vi "Mercury iTC control RUS PGG1.vi"() -> ()   [LabVIEW 2014]
uses:
  Mercury iXX/Public/Controls/Comms Transport Layer.ctl
  itc 503 box - control.ctl
  Mercury iXX/Public/Libraries/Auxiliary/Controls/AUX Device (Read).ctl
  Mercury iXX/Public/Controls/Manufacturing Data.ctl
  Mercury iXX/Public/Libraries/Auxiliary/Controls/AUX Signals (Read).ctl
  Mercury iXX/Public/Libraries/Auxiliary/Controls/AUX Device (Set).ctl
  Mercury iXX/Public/Libraries/Auxiliary/Controls/AUX Signals (Set).ctl
  Mercury iXX/Public/Libraries/Temperature/Controls/Temperature Device (Read).ctl
  Mercury iXX/Public/Libraries/Temperature/Controls/Temperature Sensor Type.ctl
  Mercury iXX/Public/Libraries/Temperature/Controls/Excitation Cluster.ctl
  Mercury iXX/Public/Libraries/Temperature/Controls/Excitation Type.ctl
  Mercury iXX/Public/Libraries/Temperature/Controls/Calibration Cluster.ctl
  Mercury iXX/Public/Libraries/Temperature/Controls/Calibration Interpolation.ctl
  Mercury iXX/Public/Libraries/Temperature/Controls/Loop Cluster.ctl
  Mercury iXX/Public/Libraries/Temperature/Controls/Temperature Signals Cluster.ctl
  itc 503 box state.ctl
  Mercury iXX/Public/Libraries/Heater/Controls/Heater Device (Set).ctl
  Mercury iXX/Public/Libraries/Heater/Controls/Heater Signals Cluster.ctl
  Mercury iXX/Public/Libraries/Heater/Controls/Heater Device (Read).ctl
  Mercury iXX/Public/Controls/Response String.ctl
  Mercury iXX/Public/Controls/ISOBus Address.ctl
  Mercury iXX/Public/Controls/Unit String.ctl
  Mercury iXX/Public/Libraries/Auxiliary/Open/Open Auxiliary Device.vi
  Mercury iXX/Public/Libraries/Auxiliary/Configuration/Read/Aux Device (Read).vi
  Mercury iXX/Public/Libraries/Auxiliary/Configuration/Set/Aux Device (Set).vi
  Mercury iXX/Public/Libraries/Temperature/Open/Open Temperature Device.vi
  Mercury iXX/Public/Libraries/Temperature/Configuration/Read/Temperature Device (Read).vi
  Mercury iXX/Public/Libraries/Control Loop/Configuration/Set/Temperature Setpoint (Set).vi
  Mercury iXX/Public/Libraries/Control Loop/Configuration/Set/Heater Auto (Set).vi
  Mercury iXX/Public/Libraries/Heater/Open/Open Heater Device.vi
  Mercury iXX/Public/Libraries/Heater/Configuration/Read/Heater Device (Read).vi
  Mercury iXX/Public/Libraries/Heater/Configuration/Set/Heater Device (Set).vi
  Mercury iXX/Public/Libraries/Heater/Signals/Read/Voltage (Read).vi
  Mercury iXX/Public/Libraries/Control Loop/Configuration/Read/Temperature Setpoint (Read).vi
  Mercury iXX/Public/Libraries/Control Loop/Configuration/Read/PID (Read).vi
  Mercury iXX/Public/Libraries/Control Loop/Configuration/Set/P Value (Set).vi
  Mercury iXX/Public/Libraries/Control Loop/Configuration/Set/I Value (Set).vi
  Mercury iXX/Public/Libraries/Control Loop/Configuration/Set/D Value (Set).vi
  Mercury iXX/Public/Libraries/System.lvlib
  Mercury iXX/Mercury iXX.lvlib
  Mercury iXX/Public/Libraries/Temperature.lvlib
  Mercury iXX/Public/Libraries/Auxiliary.lvlib
  Mercury iXX/Public/Libraries/Control Loop.lvlib
  Mercury iXX/Public/Libraries/Heater.lvlib
panel:
  out "Response":T1
  out "itc box state OUT":T2
  out "Tab Control":T3(tab)
  out "Auxiliary Device Details":T4 {"Signals"."% Open" min=0.0 max=100.0 step=0.1 format="%.4f"; "Signals"."Position" max=20.0 step=1.0 format="%.4f"; "Speed" max=7 step=1; "Gear" max=7 step=1; "Temp V Err" min=0.0 max=20.0 step=0.1; "Temp Err" min=0.0 max=20.0 step=0.1; "Scaling Factor" min=0.0 max=99.0 step=0.1; "Min Flow" min=0.0 max=20.0 step=0.1}
  in  "Auxiliary Device":T7 {"Signals"."% Open" min=0.0 max=100.0 step=0.1 format="%#.1f"; "Speed" max=7 step=1; "Gear" max=7 step=1; "Temp V Err" min=0.0 max=20.0 step=0.1; "Temp Err" min=0.0 max=20.0 step=0.1; "Scaling Factor" min=0.0 max=99.0 step=0.1; "Min Flow" min=0.0 max=20.0 step=0.1}
  out "# of Instruments":i32
  out "Serial Number(s)":string[](array[string])
  out "T config Details":T9
  in  "T config Void":T9
  in  "Heater Device Void":T17
  out "Heater Config Details In":T19
  out "Temperature":dbl
  out "error out":errorcluster={"status"=TRUE, "code"=-1073807343, "source"="VISA Open in Mercury iXX.lvlib:System.lvlib:Open System.vi->Mercury iTC control RUS PGG1.vi"}
  in  "disable interaction with iTC":enum16{"disabled", "enabled"}(ring)
  in  "input":dbl=300.0
  in  "itc box action":T20=enum."read state"
  in  "Comms Layer":T21=enum."GPIB"
  in  "VISA resource name":refnum<visa-resource-name>="GPIB0::1::1::INSTR"
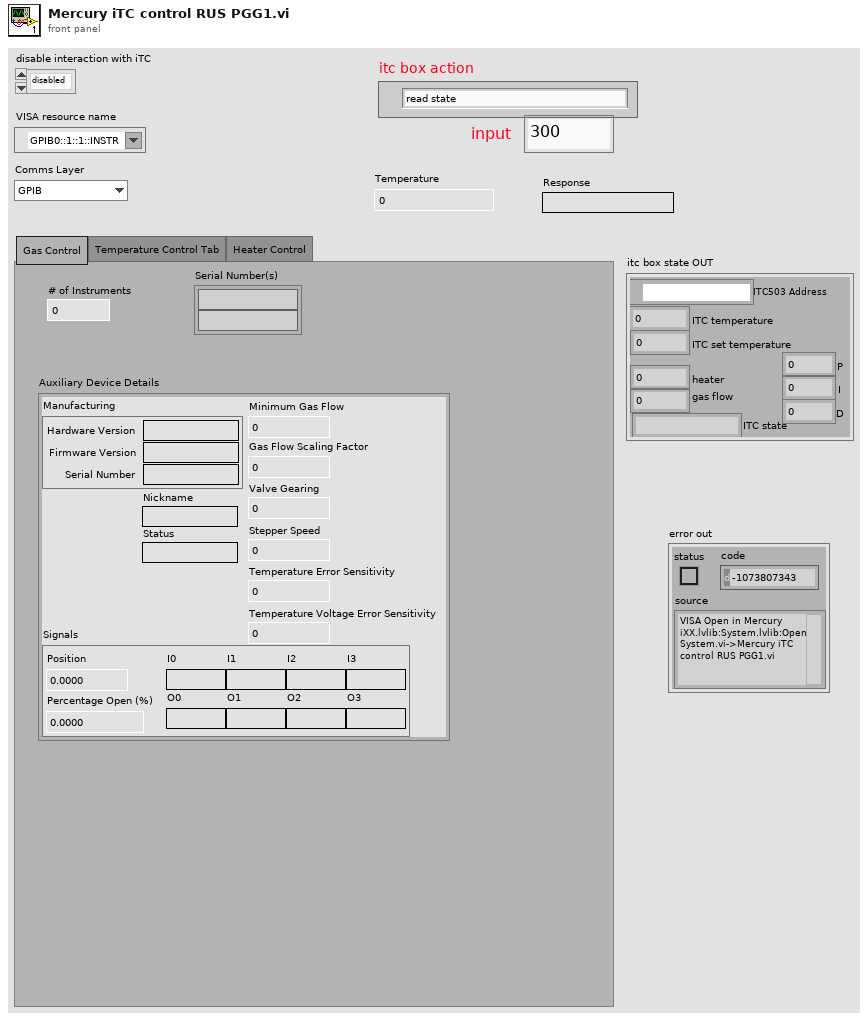
[diagram p1: front panel]
types:
  T1 = typedef "Mercury iXX.lvlib/Response String.ctl" = string
  T2 = typedef "itc 503 box state.ctl" = cluster{"ITC503 Address":refnum<visa-resource-name>, "ITC temperature":dbl, "ITC set temperature":dbl, "heater":dbl, "gas flow":dbl, "P":dbl, "D":dbl, "I":dbl, "ITC state":string, "nonzero temperature":dbl, "Magn Field (T)":dbl}
  T3 = enum32{"Gas Control", "Temperature Control Tab", "Heater Control"}
  T4 = typedef "Mercury iXX.lvlib/Auxiliary.lvlib/AUX Device (Read).ctl" = cluster{"Manufacturing":T5, "Min Flow":dbl, "Scaling Factor":dbl, "Temp Err":dbl, "Temp V Err":dbl, "Gear":u32, "Speed":u32, "Signals":T6, "Nickname":string, "Status":string}
  T5 = typedef "Mercury iXX.lvlib/Manufacturing Data.ctl" = cluster{"Hardware Version":string, "Firmware Version":string, "Serial Number":string}
  T6 = typedef "Mercury iXX.lvlib/Auxiliary.lvlib/AUX Signals (Read).ctl" = cluster{"Position":dbl, "% Open":dbl, "I0":string, "I1":string, "I2":string, "I3":string, "O0":string, "O1":string, "O2":string, "O3":string}
  T7 = typedef "Mercury iXX.lvlib/Auxiliary.lvlib/AUX Device (Set).ctl" = cluster{"Min Flow":dbl, "Scaling Factor":dbl, "Temp Err":dbl, "Temp V Err":dbl, "Gear":u32, "Speed":u32, "Signals":T8}
  T8 = typedef "Mercury iXX.lvlib/Auxiliary.lvlib/AUX Signals (Set).ctl" = cluster{"% Open":dbl}
  T9 = typedef "Mercury iXX.lvlib/Temperature.lvlib/Temperature Device (Read).ctl" = cluster{"Manufacturing":T5, "Temperature Sensor Type":T10, "Excitation":T11, "Calibration":T13, "Control Loop":T15, "Temperature Signals":T16, "Nickname":string, "Status":string}
  T10 = typedef "Mercury iXX.lvlib/Temperature.lvlib/Temperature Sensor Type.ctl" = string
  T11 = typedef "Mercury iXX.lvlib/Temperature.lvlib/Excitation Cluster.ctl" = cluster{"Excitation Type":T12, "Magnitude":string}
  T12 = typedef "Mercury iXX.lvlib/Temperature.lvlib/Excitation Type.ctl" = string
  T13 = typedef "Mercury iXX.lvlib/Temperature.lvlib/Calibration Cluster.ctl" = cluster{"Filename":string, "Interpolation":T14, "Scaling Factor":string, "Offset Factor":string, "Hot Limit":string, "Cold Limit":string, "Last Calibration":string, "Reference":string}
  T14 = typedef "Mercury iXX.lvlib/Temperature.lvlib/Calibration Interpolation.ctl" = string
  T15 = typedef "Mercury iXX.lvlib/Temperature.lvlib/Loop Cluster.ctl" = cluster{"Heater":string, "Auxiliary":string, "Heater Auto":string, "Percentage Heat":string, "Temperature Set Point":string, "PID Auto (from file)":string, "P Value":string, "I Value":string, "D Value":string, "Auto PID Table Filename":string, "Flow Auto":string, "Target Heater Table":string, "Sweep mode":string, "Sweep Table Filename":string, "Percentage Flow":string}
  T16 = typedef "Mercury iXX.lvlib/Temperature.lvlib/Temperature Signals Cluster.ctl" = cluster{"Voltage":string, "Current":string, "Power":string, "Resistance":string, "Temperature":string, "Sensitivity":string, "Reference":string}
  T17 = typedef "Mercury iXX.lvlib/Heater.lvlib/Heater Device (Set).ctl" = cluster{"Nickname":string, "Voltage Limit":string, "Nominal Resistance":string, "Maximum Power":string, "Heater Signals":T18}
  T18 = typedef "Mercury iXX.lvlib/Heater.lvlib/Heater Signals Cluster.ctl" = cluster{"Voltage":string, "Current":string, "Power":string}
  T19 = typedef "Mercury iXX.lvlib/Heater.lvlib/Heater Device (Read).ctl" = cluster{"Manufacturing":T5, "Nickname":string, "Voltage Limit":string, "Nominal Resistance":string, "Maximum Power":string, "Heater Signals":T18, "Status":string}
  T20 = typedef "itc 503 box - control.ctl" = enum16{"heater manual and zero", "heater auto", "upload D", "upload I", "upload P", "shut off", "init", "read sweep table", "disable", "enable", "read state", "set gas to", "stop sweep", "start sweep", "test", "set temperature to", "write sweep table", "-void", "set heater to"}
  T21 = typedef "Mercury iXX.lvlib/Comms Transport Layer.ctl" = enum16{"Ethernet TCP/IP", "USB", "ISOBus - RS-232", "GPIB"}
  T22 = typedef "Mercury iXX.lvlib/ISOBus Address.ctl" = i32
  T23 = typedef "Mercury iXX.lvlib/Mercury Reference.ctl" = cluster{"Comms":refnum<visa-resource-name>, "Device ID":string[], "Comms Layer":T21, "Command":string, "Query reference":T24}
  T24 = typedef "Mercury iXX.lvlib/Query Dynamic Reference.ctl" = refnum<vi>
  T25 = typedef "Mercury iXX.lvlib/Unit String.ctl" = string
  T26 = typedef "Mercury iXX.lvlib/Control Loop.lvlib/PID cluster.ctl" = cluster{"P":dbl, "I":dbl, "D":dbl}
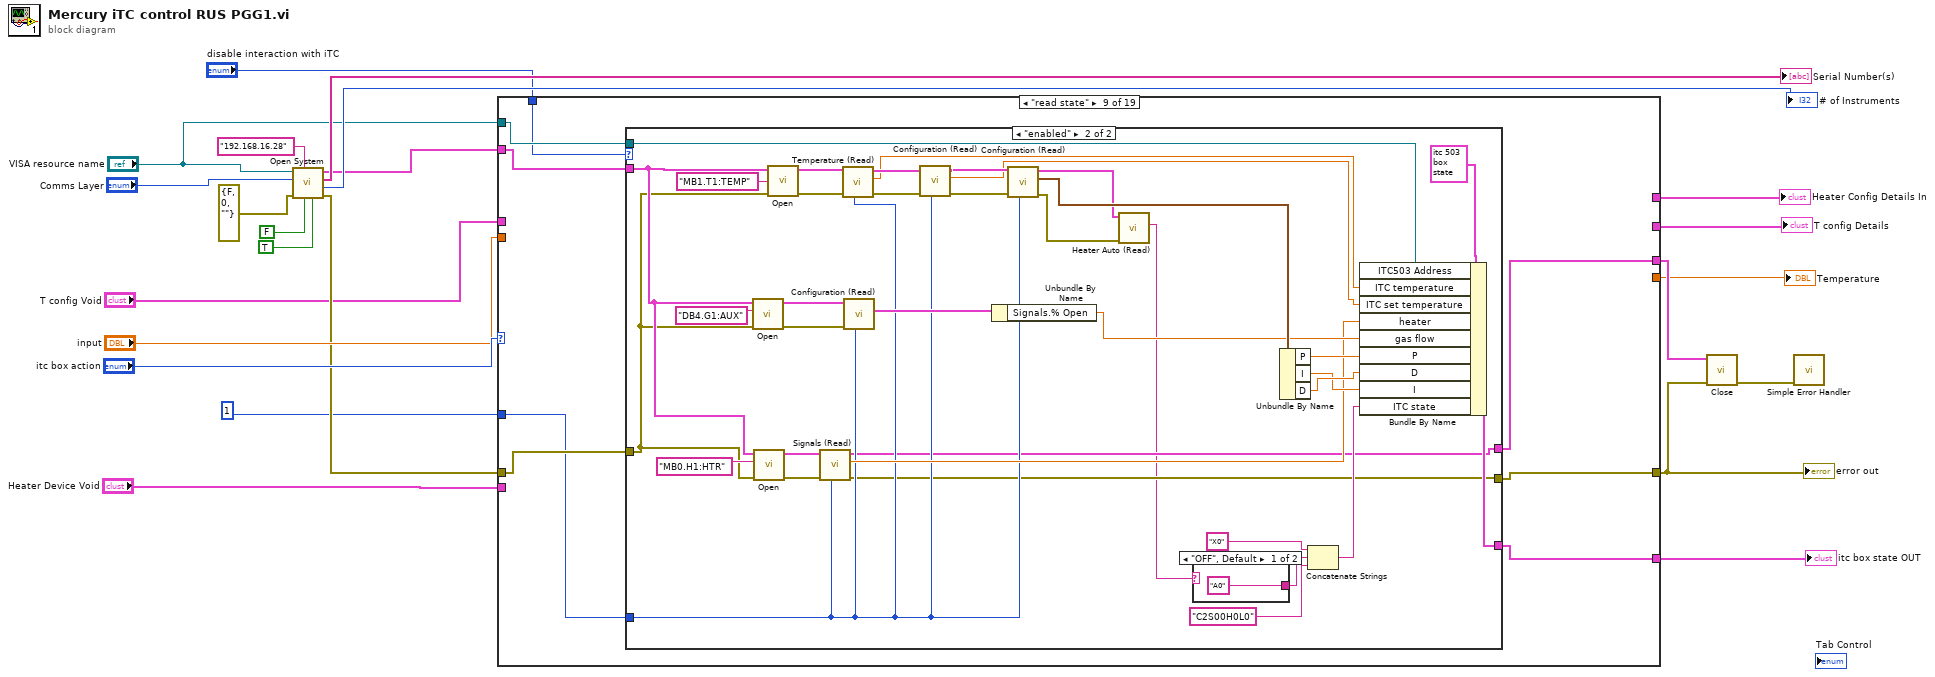
[diagram p0: block diagram]
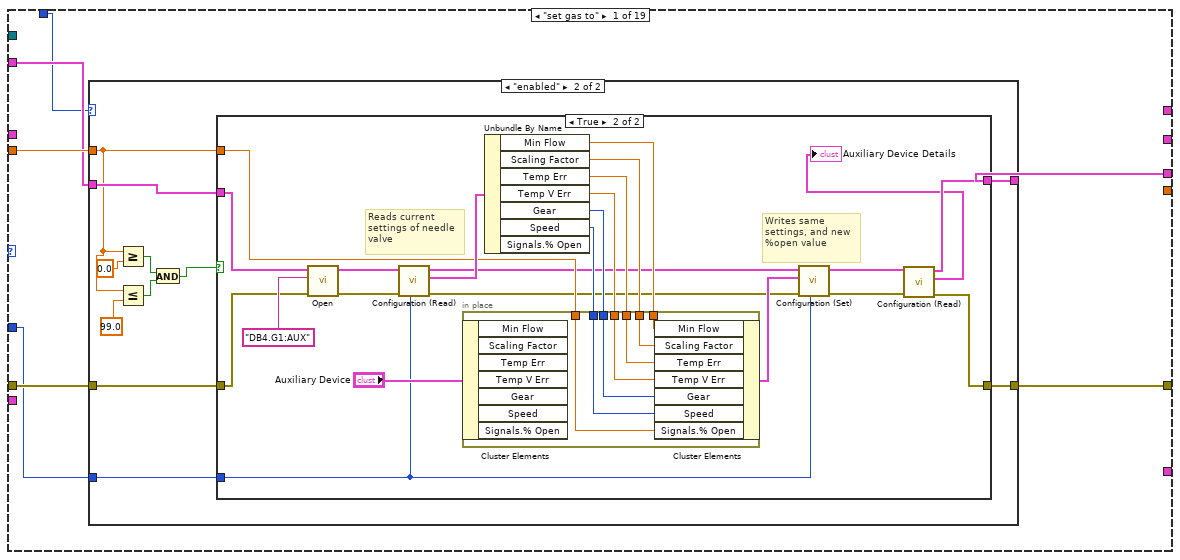
[diagram p2: hidden frame]
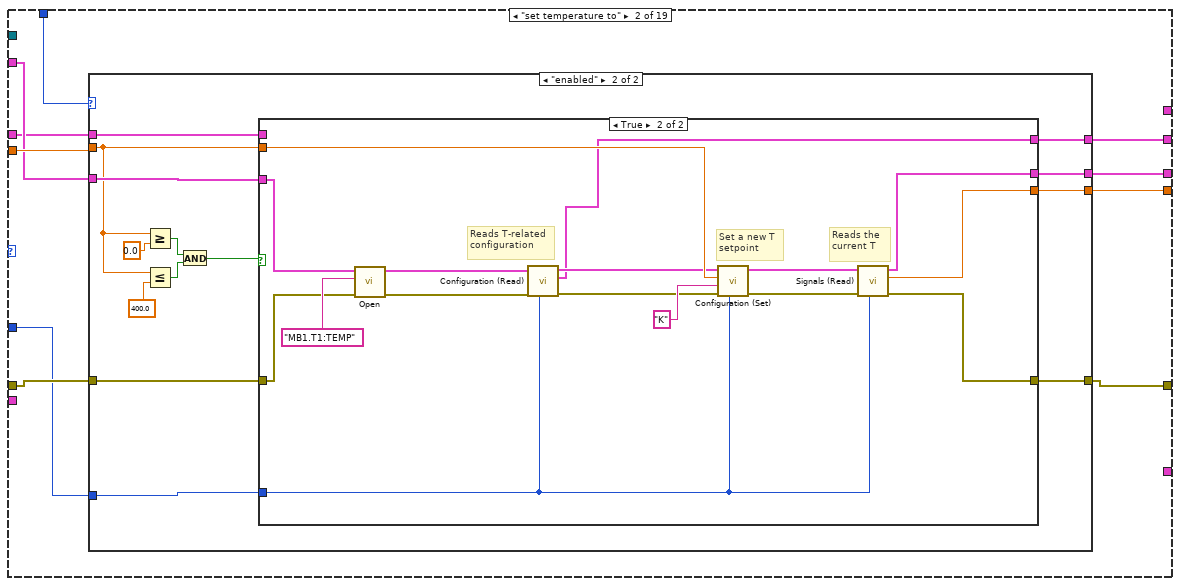
[diagram p5: hidden frame]
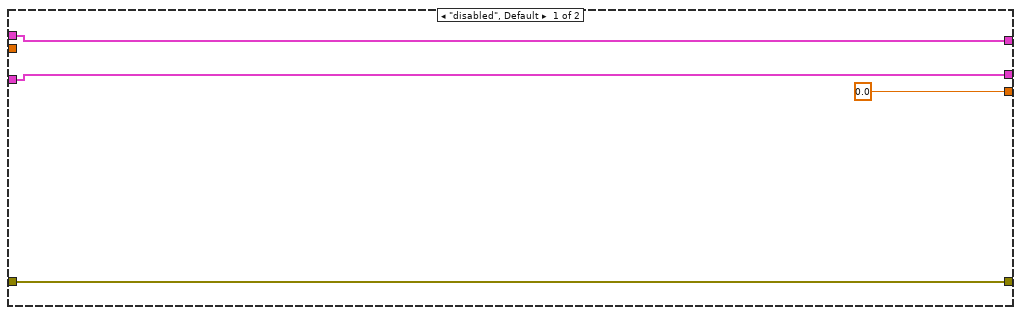
[diagram p6: hidden frame]
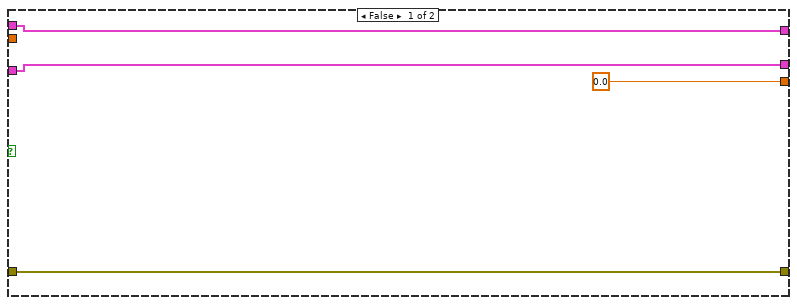
[diagram p7: hidden frame]
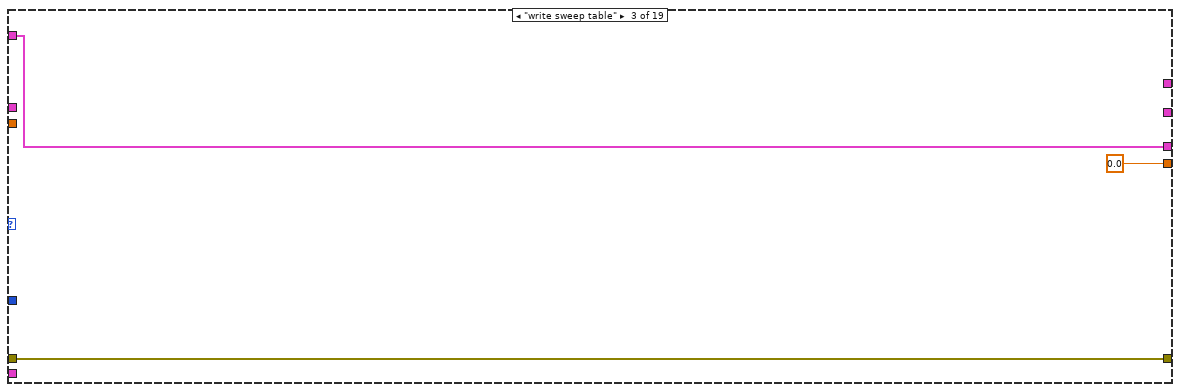
[diagram p8: hidden frame]
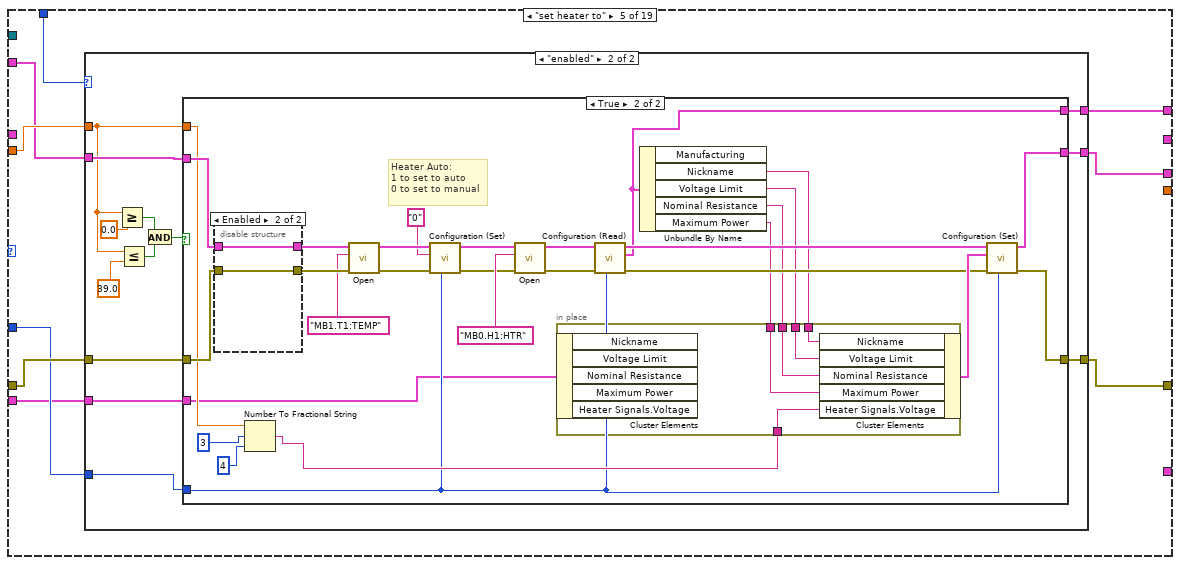
[diagram p10: hidden frame]
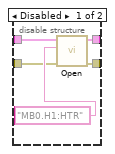
[diagram p13: hidden frame]
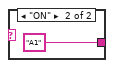
[diagram p18: hidden frame]
diagram:
  n1 = call "Open System.vi"("Clear Previous Connections (False)"=TRUE, "ID Query (True)"=FALSE, "IP Address"="192.168.16.28", "error in (no error)"=errorcluster {"status"=FALSE, "code"=0, "source"=""}, "Comms Layer"="Comms Layer", "VISA resource name"="VISA resource name") -> ("error out"=w14:errorcluster, "# of Instruments"=→"# of Instruments":i32, "Serial Number(s)"=→"Serial Number(s)":string[], "Mercury Reference Out"=w15:T23)  [unwired: 1 in, 1 out]
  n2 = case shown="\"read state\"" "itc box action" {
    tunnel: "input" -> [w30 w85 _ _ w136 _ _ _ _ _ _ _ _ _ w269 w310 w365 _ _]
    tunnel: w15 -> [w29 w84 w126 w128 w135 w197 w199 w200 w206 w252 w254 w256 w258 w260 w268 w311 w364 w408 w445]
    tunnel: w14 -> [w28 w83 w125 w127 w134 w196 w198 w201 w208 w251 w253 w255 w257 w259 w267 w313 w361 w409 w447]
    tunnel: "disable interaction with iTC" -> [w27 w81 _ _ w137 _ _ _ w203 _ _ _ _ _ w270 w309 w366 w406 w443]
    tunnel: [w26 w82 w125 w127 w132 w196 w198 w201 w205 w251 w253 w255 w257 w259 w265 w315 w360 w407 w441] -> w11
    tunnel: [w25 w80 w126 w128 w131 w197 w199 w200 w202 w252 w254 w256 w258 w260 w264 w317 w358 w405 w442] -> w10
    tunnel: [_ w79 0.0 ("Temperature") _ _ _ _ _ _ _ _ _ _ _ w263 w316 w359 _ _] -> w8
    tunnel: T22 1 ("ISOBUS address") -> [w24 w78 _ _ w133 _ _ _ w207 _ _ _ _ _ w266 w314 w362 w410 w446]
    tunnel: [_ w77 _ _ _ _ _ _ _ _ _ _ _ _ w262 w318 w357 _ _] -> w5
    tunnel: "T config Void" -> [_ w76 _ _ _ _ _ _ _ _ _ _ _ _ w261 w312 w363 _ _]
    tunnel: "VISA resource name" -> [_ _ _ _ _ _ _ _ w209 _ _ _ _ _ _ _ _ _ _]
    tunnel: [_ _ _ _ _ _ _ _ w204 _ _ _ _ _ _ _ _ _ _] -> w3
    tunnel: "Heater Device Void" -> [_ _ _ _ w130 _ _ _ _ _ _ _ _ _ _ _ _ _ w444]
    tunnel: [_ _ _ _ w129 _ _ _ _ _ _ _ _ _ _ _ _ _ w440] -> w1
    frame "set gas to" {
      n3 = case shown="\"enabled\"" w27 {
        tunnel: w30 -> [_ w34]
        tunnel: w28 -> [w32 w43]
        tunnel: [w32 w42] -> w26
        tunnel: w29 -> [w31 w41]
        tunnel: [w31 w40] -> w25
        tunnel: w24 -> [_ w33]
        frame "disabled", Default {
        }
        frame "enabled" {
          n4 = Greater Or Equal?(x=w34, y=0.0) -> (x >= y?=w36:bool)
          n5 = Less Or Equal?(x=w34, y=99.0) -> (x <= y?=w37:bool)
          n6 = And(x=w36, y=w37) -> (x .and. y?=w35:bool)
          n7 = case shown="True" w35 {
            tunnel: w43 -> [w45 w66]
            tunnel: [w45 w48] -> w42
            tunnel: w34 -> [_ w54]
            tunnel: w41 -> [w44 w67]
            tunnel: [w44 w49] -> w40
            tunnel: w33 -> [_ w51]
            frame False {
            }
            frame True {
              # "Writes same settings, and new %open value"
              # "Reads current settings of needle valve"
              n8 = call-poly "Open.vi"("error in (no error)"=w66, "Device Identifier"="DB4.G1:AUX", "Mercury Reference In"=w67) -> ("error out"=w64:errorcluster, "Mercury Reference Out"=w65:T23)  [unwired: 7 out]
              n9 = call-poly "Configuration (Read).vi"("ISOBUS address"=w51, "error in"=w64, "Mercury Reference In"=w65) -> ("error out"=w52:errorcluster, "Auxiliary Device Details"=w63:T4, "Mercury Reference Out"=w53:T23)  [unwired: 6 out]
              n10 = Unbundle By Name(w63) -> ("Min Flow"=w60:dbl, "Scaling Factor"=w59:dbl, "Temp Err"=w58:dbl, "Temp V Err"=w57:dbl, "Gear"=w56:u32, "Speed"=w55:u32)  [unwired: 1 out]
              n11 = in-place {
                in-place-border: w60 -> [w75]
                in-place-border: w59 -> [w74]
                in-place-border: w58 -> [w73]
                in-place-border: w57 -> [w72]
                in-place-border: w56 -> [w71]
                in-place-border: w55 -> [w70]
                in-place-border: w54 -> [w69]
                n12 = in-place-cluster #1("Auxiliary Device") -> ()  [unwired: 7 out]
                n13 = in-place-cluster #1("Min Flow"=w75, "Scaling Factor"=w74, "Temp Err"=w73, "Temp V Err"=w72, "Gear"=w71, "Speed"=w70, "Signals.% Open"=w69) -> (w61:T7)
              }
              n14 = call-poly "Configuration (Set).vi"("ISOBUS address"=w51, "error in"=w52, "Auxiliary Device"=w61, "Mercury Reference In"=w53) -> ("error out"=w47:errorcluster, "Mercury Reference Out"=w50:T23)  [unwired: 4 in, 2 out]
              n15 = call-poly "Configuration (Read).vi"("error in"=w47, "Mercury Reference In"=w50) -> ("error out"=w48:errorcluster, "Auxiliary Device Details"=→"Auxiliary Device Details":T4, "Mercury Reference Out"=w49:T23)  [unwired: 1 in, 6 out]
            }
          }
        }
      }
    }
    frame "set temperature to" {
      n16 = case shown="\"enabled\"" w81 {
        tunnel: w85 -> [_ w94]
        tunnel: w83 -> [w89 w102]
        tunnel: [w89 w103] -> w82
        tunnel: w84 -> [w88 w101]
        tunnel: [w88 w100] -> w80
        tunnel: [0.0 ("Temperature") w93] -> w79
        tunnel: w78 -> [_ w92]
        tunnel: [w86 w91] -> w77
        tunnel: w76 -> [w86 w90]
        frame "disabled", Default {
        }
        frame "enabled" {
          n17 = Greater Or Equal?(x=w94, y=0.0) -> (x >= y?=w96:bool)
          n18 = Less Or Equal?(x=w94, y=400.0) -> (x <= y?=w97:bool)
          n19 = And(x=w96, y=w97) -> (x .and. y?=w95:bool)
          n20 = case shown="True" w95 {
            tunnel: [w107 w120] -> w103
            tunnel: w94 -> [_ w115]
            tunnel: w102 -> [w107 w121]
            tunnel: w101 -> [w106 w122]
            tunnel: [w106 w119] -> w100
            tunnel: [0.0 ("Temperature") w118] -> w93
            tunnel: w92 -> [_ w109]
            tunnel: [w104 w108] -> w91
            tunnel: w90 -> [w104 _]
            frame False {
            }
            frame True {
              # "Reads the current T"
              # "Set a new T setpoint"
              # "Reads T-related configuration"
              n21 = call-poly "Open.vi"("error in (no error)"=w121, "Device Identifier"="MB1.T1:TEMP", "Mercury Reference In"=w122) -> ("error out"=w112:errorcluster, "Mercury Reference Out"=w113:T23)  [unwired: 7 out]
              n22 = call-poly "Configuration (Read).vi"("ISOBUS address"=w109, "error in"=w112, "Mercury Reference In"=w113) -> ("error out"=w111:errorcluster, "Device Details"=w108:T9, "Mercury Reference Out"=w110:T23)  [unwired: 6 out]
              n23 = call-poly "Configuration (Set).vi"("ISOBUS address"=w109, "error in"=w111, "Unit"=T25 "K", "Temperature setpoint"=w115, "Mercury Reference In"=w110) -> ("error out"=w116:errorcluster, "Mercury Reference Out"=w117:T23)  [unwired: 3 in, 2 out]
              n24 = call-poly "Signals (Read).vi"("ISOBUS address"=w109, "error in"=w116, "Mercury Reference In"=w117) -> ("error out"=w120:errorcluster, "Temperature"=w118:dbl, "Mercury Reference Out"=w119:T23)  [unwired: 6 out]
            }
          }
        }
      }
    }
    frame "write sweep table" {
    }
    frame "-void" {
    }
    frame "set heater to" {
      n25 = case shown="\"enabled\"" w137 {
        tunnel: w136 -> [_ w143]
        tunnel: w134 -> [w139 w151]
        tunnel: [w139 w152] -> w132
        tunnel: w135 -> [w138 w150]
        tunnel: [w138 w149] -> w131
        tunnel: w133 -> [_ w142]
        tunnel: w130 -> [_ w141]
        tunnel: [_ w140] -> w129
        frame "disabled", Default {
        }
        frame "enabled" {
          n26 = Greater Or Equal?(x=w143, y=0.0) -> (x >= y?=w145:bool)
          n27 = Less Or Equal?(x=w143, y=39.0) -> (x <= y?=w146:bool)
          n28 = And(x=w145, y=w146) -> (x .and. y?=w144:bool)
          n29 = case shown="True" w144 {
            tunnel: [w154 w170] -> w152
            tunnel: w143 -> [_ w172]
            tunnel: w151 -> [w154 w182]
            tunnel: w150 -> [w153 w183]
            tunnel: [w153 w169] -> w149
            tunnel: w142 -> [_ w166]
            tunnel: w141 -> [_ w156]
            tunnel: [_ w155] -> w140
            frame False {
            }
            frame True {
              # "Heater Auto:\n1 to set to auto\n0 to set to manual"
              n30 = disable-structure shown="Enabled" {
                disable-tunnel: w183 -> [w187 w190]
                disable-tunnel: w182 -> [w186 w189]
                disable-tunnel: [w185 w190] -> w168
                disable-tunnel: [w184 w189] -> w167
                frame Disabled {
                  n31 = call-poly "Open.vi"("error in (no error)"=w186, "Device Identifier"="MB0.H1:HTR", "Mercury Reference In"=w187) -> ("error out"=w184:errorcluster, "Mercury Reference Out"=w185:T23)  [unwired: 7 out]
                }
                frame Enabled {
                }
              }
              n32 = Number To Fractional String(number=w172, width (-)=i16 3, precision (6)=i16 4) -> (F-format string=w174:string)  [unwired: 1 in]
              n33 = call-poly "Open.vi"("error in (no error)"=w167, "Device Identifier"="MB1.T1:TEMP", "Mercury Reference In"=w168) -> ("error out"=w163:errorcluster, "Mercury Reference Out"=w164:T23)  [unwired: 7 out]
              n34 = call-poly "Configuration (Set).vi"("ISOBUS address"=w166, "error in"=w163, "Heater Auto"="0", "Mercury Reference In"=w164) -> ("error out"=w157:errorcluster, "Mercury Reference Out"=w160:T23)  [unwired: 4 in, 2 out]
              n35 = call-poly "Open.vi"("error in (no error)"=w157, "Device Identifier"="MB0.H1:HTR", "Mercury Reference In"=w160) -> ("error out"=w158:errorcluster, "Mercury Reference Out"=w159:T23)  [unwired: 7 out]
              n36 = call-poly "Configuration (Read).vi"("ISOBUS address"=w166, "error in"=w158, "Mercury Reference In"=w159) -> ("error out"=w180:errorcluster, "Device Details"=w155:T19, "Mercury Reference Out"=w179:T23)  [unwired: 6 out]
              n37 = Unbundle By Name(w155) -> ("Nickname"=w178:string, "Voltage Limit"=w177:string, "Nominal Resistance"=w176:string, "Maximum Power"=w175:string)  [unwired: 1 out]
              n38 = in-place {
                in-place-border: w178 -> [w195]
                in-place-border: w177 -> [w194]
                in-place-border: w176 -> [w193]
                in-place-border: w175 -> [w192]
                in-place-border: w174 -> [w191]
                n39 = in-place-cluster #2(w156) -> ()  [unwired: 5 out]
                n40 = in-place-cluster #2("Nickname"=w195, "Voltage Limit"=w194, "Nominal Resistance"=w193, "Maximum Power"=w192, "Heater Signals.Voltage"=w191) -> (w181:T17)
              }
              n41 = call-poly "Configuration (Set).vi"("ISOBUS address"=w166, "error in"=w180, "Heater Device Settings"=w181, "Mercury Reference In"=w179) -> ("error out"=w170:errorcluster, "Mercury Reference Out"=w169:T23)  [unwired: 4 in, 2 out]
            }
          }
        }
      }
    }
    frame "stop sweep" {
    }
    frame "start sweep" {
    }
    frame "test" {
    }
    frame "read state" {
      n42 = case shown="\"enabled\"" w203 {
        tunnel: [_ w246] -> w204
        tunnel: w208 -> [w211 w218]
        tunnel: [w211 w215] -> w205
        tunnel: w206 -> [w210 w219]
        tunnel: w209 -> [_ w226]
        tunnel: w207 -> [_ w217]
        tunnel: [w210 w216] -> w202
        frame "disabled", Default {
        }
        frame "enabled" {
          n43 = call-poly "Open.vi"("error in (no error)"=w218, "Device Identifier"="DB4.G1:AUX", "Mercury Reference In"=w219) -> ("error out"=w243:errorcluster, "Mercury Reference Out"=w244:T23)  [unwired: 7 out]
          n44 = call-poly "Open.vi"("error in (no error)"=w218, "Device Identifier"="MB0.H1:HTR", "Mercury Reference In"=w219) -> ("error out"=w239:errorcluster, "Mercury Reference Out"=w240:T23)  [unwired: 7 out]
          n45 = call-poly "Open.vi"("error in (no error)"=w218, "Device Identifier"="MB1.T1:TEMP", "Mercury Reference In"=w219) -> ("error out"=w220:errorcluster, "Mercury Reference Out"=w221:T23)  [unwired: 7 out]
          n46 = call-poly "Signals (Read).vi"("ISOBUS address"=w217, "error in"=w239, "Mercury Reference In"=w240) -> ("error out"=w215:errorcluster, "Voltage"=w227:dbl, "Mercury Reference Out"=w216:T23)  [unwired: 6 out]
          n47 = call "Temperature (Read).vi"("ISOBUS address"=w217, "error in"=w220, "Mercury Reference In"=w221) -> ("error out"=w238:errorcluster, "Temperature"=w234:dbl, "Mercury Reference Out"=w237:T23)  [unwired: 4 in, 2 out]
          n48 = call-poly "Configuration (Read).vi"("ISOBUS address"=w217, "error in"=w243, "Mercury Reference In"=w244) -> ("Auxiliary Device Details"=w242:T4)  [unwired: 8 out]
          n49 = call-poly "Configuration (Read).vi"("ISOBUS address"=w217, "error in"=w238, "Mercury Reference In"=w237) -> ("error out"=w235:errorcluster, "Temperature Setpoint"=w233:dbl, "Mercury Reference Out"=w236:T23)  [unwired: 6 out]
          n50 = Unbundle By Name(w242) -> ("Signals.% Open"=w228:dbl)
          n51 = call-poly "Configuration (Read).vi"("ISOBUS address"=w217, "error in"=w235, "Mercury Reference In"=w236) -> ("error out"=w213:errorcluster, "PID"=w232:T26, "Mercury Reference Out"=w214:T23)  [unwired: 6 out]
          n52 = call "Heater Auto (Read).vi"("error in"=w213, "Mercury Reference In"=w214) -> ("Heater Auto"=w212:string)  [unwired: 6 in, 3 out]
          n53 = case shown="\"OFF\", Default" w212 {
            tunnel: ["A0" "A1"] -> w225
            frame "OFF", Default {
            }
            frame "ON" {
            }
          }
          n54 = Unbundle By Name(w232) -> ("P"=w231:dbl, "I"=w229:dbl, "D"=w230:dbl)
          n55 = Concatenate Strings("X0", w225, "C2S00H0L0") -> (w222:string)
          n56 = Bundle By Name(cluster=T2 {"ITC503 Address"="GPIB0::15::INSTR", "ITC temperature"=0.0, "ITC set temperature"=0.0, "heater"=0.0, "gas flow"=0.0, "P"=0.0, "D"=0.0, "I"=0.0, "ITC state"="", "nonzero temperature"=0.0, "Magn Field (T)"=0.0} ("itc box state OUT"), "ITC503 Address"=w226, "ITC temperature"=w234, "ITC set temperature"=w233, "heater"=w227, "gas flow"=w228, "P"=w231, "D"=w230, "I"=w229, "ITC state"=w222) -> (w246:T2)
        }
      }
    }
    frame "enable" {
    }
    frame "disable" {
    }
    frame "read sweep table" {
    }
    frame "init" {
    }
    frame "shut off" {
    }
    frame "upload P" {
      n57 = case shown="\"enabled\"" w270 {
        tunnel: w269 -> [_ w277]
        tunnel: w267 -> [w274 w287]
        tunnel: [w274 w288] -> w265
        tunnel: w268 -> [w273 w278]
        tunnel: [w273 w286] -> w264
        tunnel: [0.0 ("Temperature") w280] -> w263
        tunnel: w266 -> [_ w279]
        tunnel: [w271 w276] -> w262
        tunnel: w261 -> [w271 w275]
        frame "disabled", Default {
        }
        frame "enabled" {
          n58 = Greater Or Equal?(x=w277, y=0.0) -> (x >= y?=w282:bool)
          n59 = Less Or Equal?(x=w277, y=400.0) -> (x <= y?=w283:bool)
          n60 = And(x=w282, y=w283) -> (x .and. y?=w281:bool)
          n61 = case shown="True" w281 {
            tunnel: [w292 w305] -> w288
            tunnel: w277 -> [_ w300]
            tunnel: w287 -> [w292 w306]
            tunnel: w278 -> [w291 w307]
            tunnel: [w291 w304] -> w286
            tunnel: [0.0 ("Temperature") w303] -> w280
            tunnel: w279 -> [_ w294]
            tunnel: [w289 w293] -> w276
            tunnel: w275 -> [w289 _]
            frame False {
            }
            frame True {
              # "Reads the current T"
              # "Sets a new P value"
              # "Reads T-related configuration"
              n62 = call-poly "Open.vi"("error in (no error)"=w306, "Device Identifier"="MB1.T1:TEMP", "Mercury Reference In"=w307) -> ("error out"=w297:errorcluster, "Mercury Reference Out"=w298:T23)  [unwired: 7 out]
              n63 = call-poly "Configuration (Read).vi"("ISOBUS address"=w294, "error in"=w297, "Mercury Reference In"=w298) -> ("error out"=w296:errorcluster, "Device Details"=w293:T9, "Mercury Reference Out"=w295:T23)  [unwired: 6 out]
              n64 = call-poly "Configuration (Set).vi"("ISOBUS address"=w294, "error in"=w296, "Unit"=T25 "", "P Value"=w300, "Mercury Reference In"=w295) -> ("error out"=w301:errorcluster, "Mercury Reference Out"=w302:T23)  [unwired: 3 in, 2 out]
              n65 = call-poly "Signals (Read).vi"("ISOBUS address"=w294, "error in"=w301, "Mercury Reference In"=w302) -> ("error out"=w305:errorcluster, "Temperature"=w303:dbl, "Mercury Reference Out"=w304:T23)  [unwired: 6 out]
            }
          }
        }
      }
    }
    frame "upload I" {
      n66 = case shown="\"enabled\"" w309 {
        tunnel: w310 -> [_ w325]
        tunnel: w313 -> [w322 w335]
        tunnel: [w322 w336] -> w315
        tunnel: w311 -> [w321 w326]
        tunnel: [w321 w334] -> w317
        tunnel: [0.0 ("Temperature") w328] -> w316
        tunnel: w314 -> [_ w327]
        tunnel: [w319 w324] -> w318
        tunnel: w312 -> [w319 w323]
        frame "disabled", Default {
        }
        frame "enabled" {
          n67 = Greater Or Equal?(x=w325, y=0.0) -> (x >= y?=w330:bool)
          n68 = Less Or Equal?(x=w325, y=400.0) -> (x <= y?=w331:bool)
          n69 = And(x=w330, y=w331) -> (x .and. y?=w329:bool)
          n70 = case shown="True" w329 {
            tunnel: [w340 w353] -> w336
            tunnel: w325 -> [_ w348]
            tunnel: w335 -> [w340 w354]
            tunnel: w326 -> [w339 w355]
            tunnel: [w339 w352] -> w334
            tunnel: [0.0 ("Temperature") w351] -> w328
            tunnel: w327 -> [_ w342]
            tunnel: [w337 w341] -> w324
            tunnel: w323 -> [w337 _]
            frame False {
            }
            frame True {
              # "Reads the current T"
              # "Sets a new I value"
              # "Reads T-related configuration"
              n71 = call-poly "Open.vi"("error in (no error)"=w354, "Device Identifier"="MB1.T1:TEMP", "Mercury Reference In"=w355) -> ("error out"=w345:errorcluster, "Mercury Reference Out"=w346:T23)  [unwired: 7 out]
              n72 = call-poly "Configuration (Read).vi"("ISOBUS address"=w342, "error in"=w345, "Mercury Reference In"=w346) -> ("error out"=w344:errorcluster, "Device Details"=w341:T9, "Mercury Reference Out"=w343:T23)  [unwired: 6 out]
              n73 = call-poly "Configuration (Set).vi"("ISOBUS address"=w342, "error in"=w344, "Unit"=T25 "", "I Value"=w348, "Mercury Reference In"=w343) -> ("error out"=w349:errorcluster, "Mercury Reference Out"=w350:T23)  [unwired: 3 in, 2 out]
              n74 = call-poly "Signals (Read).vi"("ISOBUS address"=w342, "error in"=w349, "Mercury Reference In"=w350) -> ("error out"=w353:errorcluster, "Temperature"=w351:dbl, "Mercury Reference Out"=w352:T23)  [unwired: 6 out]
            }
          }
        }
      }
    }
    frame "upload D" {
      n75 = case shown="\"enabled\"" w366 {
        tunnel: w365 -> [_ w373]
        tunnel: w361 -> [w370 w383]
        tunnel: [w370 w384] -> w360
        tunnel: w364 -> [w369 w374]
        tunnel: [w369 w382] -> w358
        tunnel: [0.0 ("Temperature") w376] -> w359
        tunnel: w362 -> [_ w375]
        tunnel: [w367 w372] -> w357
        tunnel: w363 -> [w367 w371]
        frame "disabled", Default {
        }
        frame "enabled" {
          n76 = Greater Or Equal?(x=w373, y=0.0) -> (x >= y?=w378:bool)
          n77 = Less Or Equal?(x=w373, y=400.0) -> (x <= y?=w379:bool)
          n78 = And(x=w378, y=w379) -> (x .and. y?=w377:bool)
          n79 = case shown="True" w377 {
            tunnel: [w388 w401] -> w384
            tunnel: w373 -> [_ w396]
            tunnel: w383 -> [w388 w402]
            tunnel: w374 -> [w387 w403]
            tunnel: [w387 w400] -> w382
            tunnel: [0.0 ("Temperature") w399] -> w376
            tunnel: w375 -> [_ w390]
            tunnel: [w385 w389] -> w372
            tunnel: w371 -> [w385 _]
            frame False {
            }
            frame True {
              # "Reads the current T"
              # "Sets a new D value"
              # "Reads T-related configuration"
              n80 = call-poly "Open.vi"("error in (no error)"=w402, "Device Identifier"="MB1.T1:TEMP", "Mercury Reference In"=w403) -> ("error out"=w393:errorcluster, "Mercury Reference Out"=w394:T23)  [unwired: 7 out]
              n81 = call-poly "Configuration (Read).vi"("ISOBUS address"=w390, "error in"=w393, "Mercury Reference In"=w394) -> ("error out"=w392:errorcluster, "Device Details"=w389:T9, "Mercury Reference Out"=w391:T23)  [unwired: 6 out]
              n82 = call-poly "Configuration (Set).vi"("ISOBUS address"=w390, "error in"=w392, "Unit"=T25 "", "D Value"=w396, "Mercury Reference In"=w391) -> ("error out"=w397:errorcluster, "Mercury Reference Out"=w398:T23)  [unwired: 3 in, 2 out]
              n83 = call-poly "Signals (Read).vi"("ISOBUS address"=w390, "error in"=w397, "Mercury Reference In"=w398) -> ("error out"=w401:errorcluster, "Temperature"=w399:dbl, "Mercury Reference Out"=w400:T23)  [unwired: 6 out]
            }
          }
        }
      }
    }
    frame "heater auto" {
      n84 = case shown="\"enabled\"" w406 {
        tunnel: w409 -> [w412 w417]
        tunnel: [w412 w418] -> w407
        tunnel: w408 -> [w411 w414]
        tunnel: [w411 w416] -> w405
        tunnel: w410 -> [_ w415]
        frame "disabled", Default {
        }
        frame "enabled" {
          n85 = case shown="True" TRUE {
            tunnel: [w420 w425] -> w418
            tunnel: w417 -> [w420 w431]
            tunnel: w414 -> [w419 w432]
            tunnel: [w419 w424] -> w416
            tunnel: w415 -> [_ w422]
            frame False {
            }
            frame True {
              # "Heater Auto:\n1 to set to auto\n0 to set to manual"
              n86 = disable-structure shown="Enabled" {
                disable-tunnel: w432 -> [w436 w439]
                disable-tunnel: w431 -> [w435 w438]
                disable-tunnel: [w434 w439] -> w429
                disable-tunnel: [w433 w438] -> w428
                frame Disabled {
                  n87 = call-poly "Open.vi"("error in (no error)"=w435, "Device Identifier"="MB0.H1:HTR", "Mercury Reference In"=w436) -> ("error out"=w433:errorcluster, "Mercury Reference Out"=w434:T23)  [unwired: 7 out]
                }
                frame Enabled {
                }
              }
              n88 = call-poly "Open.vi"("error in (no error)"=w428, "Device Identifier"="MB1.T1:TEMP", "Mercury Reference In"=w429) -> ("error out"=w426:errorcluster, "Mercury Reference Out"=w427:T23)  [unwired: 7 out]
              n89 = call-poly "Configuration (Set).vi"("ISOBUS address"=w422, "error in"=w426, "Heater Auto"="1", "Mercury Reference In"=w427) -> ("error out"=w425:errorcluster, "Response"=→"Response":T1, "Mercury Reference Out"=w424:T23)  [unwired: 4 in, 1 out]
            }
          }
        }
      }
    }
    frame "heater manual and zero" {
      n90 = case shown="\"enabled\"" w443 {
        tunnel: w447 -> [w449 w456]
        tunnel: [w449 w457] -> w441
        tunnel: w445 -> [w448 w455]
        tunnel: [w448 w454] -> w442
        tunnel: w446 -> [_ w453]
        tunnel: w444 -> [_ w451]
        tunnel: [_ w450] -> w440
        frame "disabled", Default {
        }
        frame "enabled" {
          n91 = case shown="True" TRUE {
            tunnel: [w459 w476] -> w457
            tunnel: w456 -> [w459 w484]
            tunnel: w455 -> [w458 w485]
            tunnel: [w458 w475] -> w454
            tunnel: w453 -> [_ w472]
            tunnel: w451 -> [_ w461]
            tunnel: [_ w460] -> w450
            frame False {
            }
            frame True {
              # "Heater Auto:\n1 to set to auto\n0 to set to manual"
              n92 = disable-structure shown="Enabled" {
                disable-tunnel: w485 -> [w489 w492]
                disable-tunnel: w484 -> [w488 w491]
                disable-tunnel: [w487 w492] -> w474
                disable-tunnel: [w486 w491] -> w473
                frame Disabled {
                  n93 = call-poly "Open.vi"("error in (no error)"=w488, "Device Identifier"="MB0.H1:HTR", "Mercury Reference In"=w489) -> ("error out"=w486:errorcluster, "Mercury Reference Out"=w487:T23)  [unwired: 7 out]
                }
                frame Enabled {
                }
              }
              n94 = call-poly "Open.vi"("error in (no error)"=w473, "Device Identifier"="MB1.T1:TEMP", "Mercury Reference In"=w474) -> ("error out"=w469:errorcluster, "Mercury Reference Out"=w470:T23)  [unwired: 7 out]
              n95 = call-poly "Configuration (Set).vi"("ISOBUS address"=w472, "error in"=w469, "Heater Auto"="0", "Mercury Reference In"=w470) -> ("error out"=w463:errorcluster, "Mercury Reference Out"=w466:T23)  [unwired: 4 in, 2 out]
              n96 = call-poly "Open.vi"("error in (no error)"=w463, "Device Identifier"="MB0.H1:HTR", "Mercury Reference In"=w466) -> ("error out"=w464:errorcluster, "Mercury Reference Out"=w465:T23)  [unwired: 7 out]
              n97 = call-poly "Configuration (Read).vi"("ISOBUS address"=w472, "error in"=w464, "Mercury Reference In"=w465) -> ("error out"=w482:errorcluster, "Device Details"=w460:T19, "Mercury Reference Out"=w481:T23)  [unwired: 6 out]
              n98 = Unbundle By Name(w460) -> ("Nickname"=w480:string, "Voltage Limit"=w479:string, "Nominal Resistance"=w478:string, "Maximum Power"=w477:string)  [unwired: 1 out]
              n99 = in-place {
                in-place-border: w480 -> [w497]
                in-place-border: w479 -> [w496]
                in-place-border: w478 -> [w495]
                in-place-border: w477 -> [w494]
                in-place-border: "0" -> [w493]
                n100 = in-place-cluster #3(w461) -> ()  [unwired: 5 out]
                n101 = in-place-cluster #3("Nickname"=w497, "Voltage Limit"=w496, "Nominal Resistance"=w495, "Maximum Power"=w494, "Heater Signals.Voltage"=w493) -> (w483:T17)
              }
              n102 = call-poly "Configuration (Set).vi"("ISOBUS address"=w472, "error in"=w482, "Heater Device Settings"=w483, "Mercury Reference In"=w481) -> ("error out"=w476:errorcluster, "Mercury Reference Out"=w475:T23)  [unwired: 4 in, 2 out]
            }
          }
        }
      }
    }
  }
  "error out" <- w11
  "Temperature" <- w8
  "T config Details" <- w5
  "itc box state OUT" <- w3
  "Heater Config Details In" <- w1
  n103 = call "Close.vi"("error in (no error)"=w11, "Mercury Reference"=w10) -> ("error out"=w12:errorcluster)  [unwired: 9 out]
  n104 = call <vilib>:"Simple Error Handler.vi"("error in (no error)"=w12) -> ()  [unwired: 1 in, 8 out]
